vi "WheelShooter Shoot(Aimbot).vi"(4 "VisionPrepButton":bool, 6 "LowerButton":bool, 7 "Override Data":T1={"SpinupDuration(10ms)"=100, "ShotDuration(10ms)"=100, "PowerScale"=1.0, "AngleShift"=0}, 8 "error in":errorcluster, 9 "Collection Trigger":bool, 10 "Vision Distance":dbl, 11 "Trigger":bool) -> (0 "error out":errorcluster, 2 "LaunchSpeed(t/100ms)":dbl, 3 "AngleMotorPosition(t)":dbl)   [LabVIEW 2015]
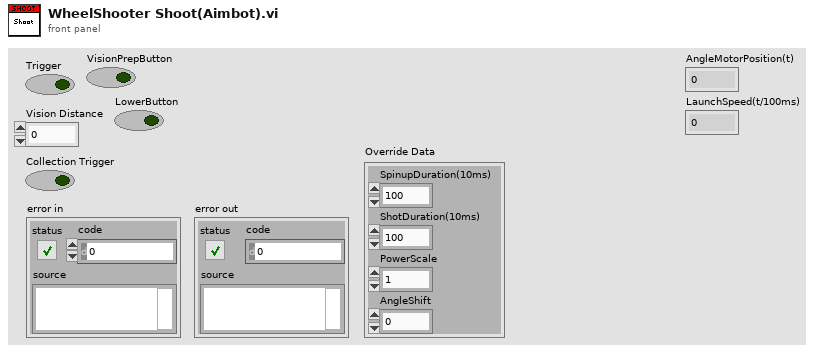
[diagram p1: front panel]
types:
  T1 = cluster{"SpinupDuration(10ms)":i32, "ShotDuration(10ms)":i32, "PowerScale":dbl, "AngleShift":i32}
  T2 = typedef "Firing Cluster.ctl" = cluster{"error":errorcluster, "AngleMotorRefnum":T3, "LeftWheelRefnum":T3, "RightWheelRefnum":T3, "PushSolenoidRefnum":T10, "AngleMotorPosition(t)":dbl, "LaunchSpeed(t/100ms)":dbl, "CollectSpeed(t/100ms)":dbl, "SpinupDuration(10ms)":i32, "ShotDuration(10ms)":i32, "PowerScale":dbl, "AngleShift":i32, "VisionPrepAngle":dbl}
  T3 = typedef "WPI_MotorControlDeviceRef.ctl" = cluster{"DeviceStatus":errorcluster, "Type":T4, "PWM":cluster{"PWM Channel":T5, "DeadBand":T6}, "CAN":cluster{"Device Number":u8, "Control Mode":T7, "Semaphore":T8, "Max Vout":dbl, "TalonSRX Control Mode":T9}, "Invert":bool}
  T4 = typedef "WPI_MotorControlType.ctl" = enum16{"PWM", "CAN", "CANTalonSRX"}
  T5 = typedef "FPGA_DIOPWMChannel.ctl" = enum8{"PWM 0", "PWM 1", "PWM 2", "PWM 3", "PWM 4", "PWM 5", "PWM 6", "PWM 7", "PWM 8", "PWM 9", "PWM MXP 0", "PWM MXP 1", "PWM MXP 2", "PWM MXP 3", "PWM MXP 4", "PWM MXP 5", "PWM MXP 6", "PWM MXP 7", "PWM MXP 8", "PWM MXP 9", "Invalid"}
  T6 = typedef "WPI_PWMDeadband.ctl" = cluster{"Name":string, "maxPositivePwm":i32, "minPositivePwm":i32, "centerPwm":i32, "maxNegativePwm":i32, "minNegativePwm":i32, "angularRange":u16}
  T7 = typedef "WPI_CANJaguar_ControlMode.ctl" = enum8{"Percent VBus", "Current", "Speed", "Position", "Voltage"}
  T8 = typedef "Semaphore RefNum" = refnum<k1>
  T9 = typedef "WPI_CANTalonSRX_APIControlMode.ctl" = enum8{"Percent VBus", "Speed", "Position", "Slave", "Unchanged / Invalid", "Voltage Compensation", "Current", "Motion Profile"}
  T10 = typedef "WPI_SolenoidDevRef.ctl" = cluster{"DevStatus":errorcluster, "Pneumatics Control Module":u8, "Forward Solenoid Channel":T11, "Reverse Solenoid Channel":T11}
  T11 = typedef "WPI_SolenoidChannel.ctl" = enum8{"Solenoid 0", "Solenoid 1", "Solenoid 2", "Solenoid 3", "Solenoid 4", "Solenoid 5", "Solenoid 6", "Solenoid 7", "Invalid"}
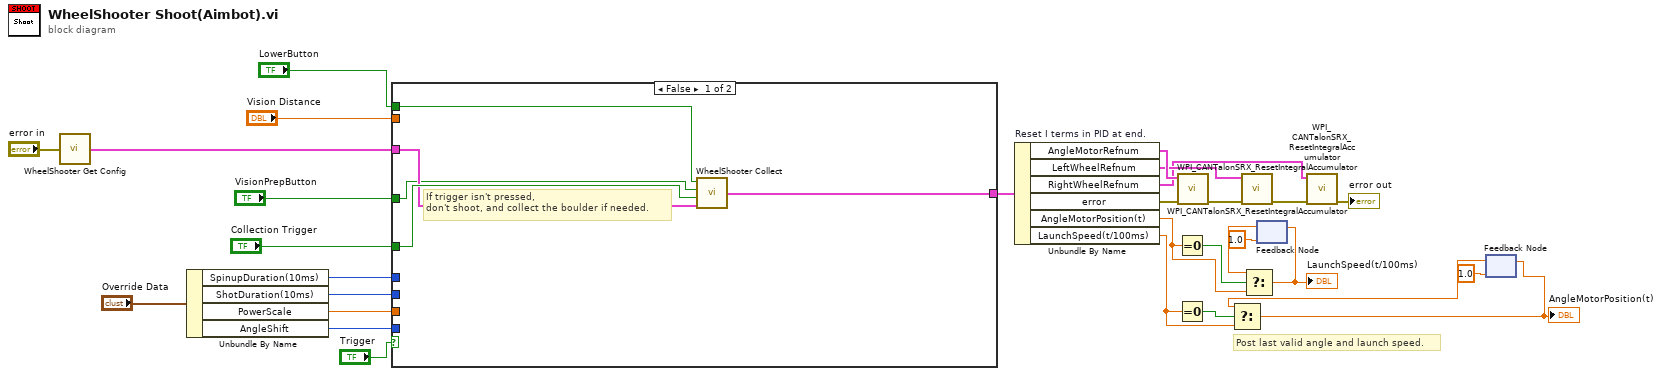
[diagram p0: block diagram]
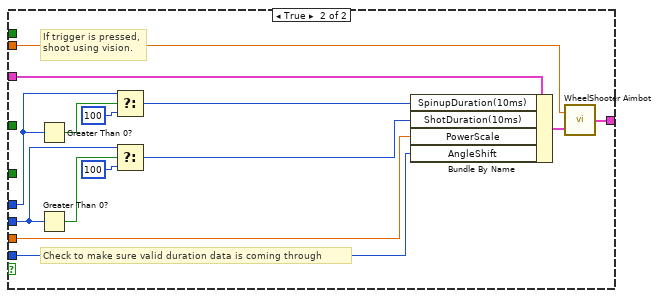
[diagram p2: hidden frame]
diagram:
  # "Post last valid angle and launch speed."
  n1 = call "WheelShooter Get Config.vi"("error in"="error in") -> (0:w24:T2)
  n2 = Unbundle By Name("Override Data") -> ("SpinupDuration(10ms)"=w6:i32, "ShotDuration(10ms)"=w5:i32, "PowerScale"=w4:dbl, "AngleShift"=w3:i32)
  n3 = case shown="False" "Trigger" {
    tunnel: [w33 w49] -> w19
    tunnel: "Vision Distance" -> [_ w48]
    tunnel: "Collection Trigger" -> [w35 _]
    tunnel: w24 -> [w34 w47]
    tunnel: w5 -> [_ w42]
    tunnel: w6 -> [_ w37]
    tunnel: w4 -> [_ w45]
    tunnel: w3 -> [_ w44]
    tunnel: "LowerButton" -> [w32 _]
    tunnel: "VisionPrepButton" -> [w31 _]
    frame False {
      # "If trigger isn't pressed,\ndon't shoot, and collect the boulder if needed."
      n4 = call "WheelShooter Collect.vi"("Firing Data"=w34, "CollectionTrigger"=w35, "VisionPrepButton"=w31, "LowerButton"=w32) -> ("Firing Data"=w33:T2)
    }
    frame True {
      # "Check to make sure valid duration data is coming through"
      # "If trigger is pressed,\nshoot using vision."
      n5 = Greater Than 0?(x=w37) -> (x > 0?=w39:bool)
      n6 = Greater Than 0?(x=w42) -> (x > 0?=w43:bool)
      n7 = Select(t=w37, s=w39, f=100) -> (s? t:f=w36:i32)
      n8 = Select(t=w42, s=w43, f=100) -> (s? t:f=w40:i32)
      n9 = Bundle By Name(cluster=w47, "SpinupDuration(10ms)"=w36, "ShotDuration(10ms)"=w40, "PowerScale"=w45, "AngleShift"=w44) -> (w46:T2)
      n10 = call "WheelShooter Aimbot.vi"("Firing Data"=w46, "Range"=w48) -> ("Firing Data out"=w49:T2)
    }
  }
  n11 = Unbundle By Name "Reset I terms in PID at end."(w19) -> ("AngleMotorRefnum"=w27:T3, "LeftWheelRefnum"=w26:T3, "RightWheelRefnum"=w25:T3, "error"=w18:errorcluster, "AngleMotorPosition(t)"=w11:dbl, "LaunchSpeed(t/100ms)"=w9:dbl)
  n12 = Equal To 0?(x=w11) -> (x = 0?=w17:bool)
  n13 = Equal To 0?(x=w9) -> (x = 0?=w14:bool)
  n14 = call <vilib>:"WPI_CANTalonSRX_ResetIntegralAccumulator.vi"("error in (no error)"=w18, "CAN Talon SRX Ref"=w27) -> ("error out"=w29:errorcluster)  [unwired: 8 in, 1 out]
  n15 = call <vilib>:"WPI_CANTalonSRX_ResetIntegralAccumulator.vi"("error in (no error)"=w29, "CAN Talon SRX Ref"=w26) -> ("error out"=w30:errorcluster)  [unwired: 8 in, 1 out]
  n16 = feedback #1(1.0) -> (w16:dbl)
  n17 = Select(t=w16, s=w17, f=w11) -> (s? t:f=w8:dbl)
  "LaunchSpeed(t/100ms)" <- w8
  n18 = feedback-in #1(w8) -> ()
  n19 = call <vilib>:"WPI_CANTalonSRX_ResetIntegralAccumulator.vi"("error in (no error)"=w30, "CAN Talon SRX Ref"=w25) -> ("error out"=→"error out":errorcluster)  [unwired: 8 in, 1 out]
  n20 = feedback #2(1.0) -> (w12:dbl)
  n21 = Select(t=w12, s=w14, f=w9) -> (s? t:f=w10:dbl)
  "AngleMotorPosition(t)" <- w10
  n22 = feedback-in #2(w10) -> ()
